vi "refresh.vi"(8 "error in (no error)":errorcluster, 10 "Engine Configuration In":refnum<class "engine configuration.lvclass">, 11 "Modbus Module editor node In":refnum<class "Modbus Module editor node.lvclass">) -> (0 "error out":errorcluster, 2 "Engine Configuration Out":refnum<class "engine configuration.lvclass">, 3 "Modbus Module editor node Out":refnum<class "Modbus Module editor node.lvclass">)   [LabVIEW 2013, in "Modbus Module editor node.lvclass"]
uses:
  Modbus Module editor node.lvclass
  <vilib>/NI/Module Execution Interface/Engine Configuration/engine configuration.lvclass
  <vilib>/NI/DCAF/Tag Editor Core/Configuration Editor/Classes/Module editor node/module editor node.lvclass
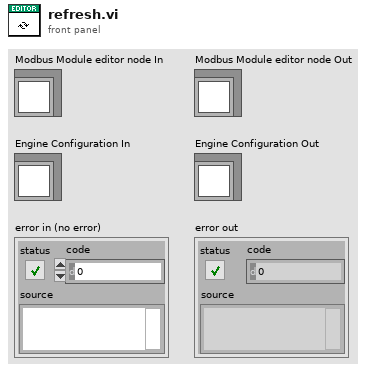
[diagram p1: front panel]
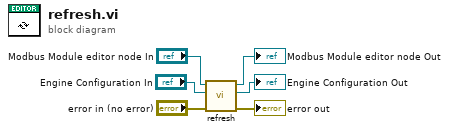
[diagram p0: block diagram]
diagram:
  n1 = call-parent "refresh.vi"("error in (no error)"="error in (no error)", "Engine Configuration In"="Engine Configuration In", "Module Editor Node In"="Modbus Module editor node In") -> ("error out"=→"error out":errorcluster, "Engine Configuration Out"=→"Engine Configuration Out":refnum<class "engine configuration.lvclass">, "Module Editor Node Out"=→"Modbus Module editor node Out":refnum<class "Modbus Module editor node.lvclass">)  [unwired: 6 in]
